vi "Convert normal string to hex string.vi"(4 "Normal String":string[](array[string])) -> (1 "Hex String":string[](array[string]))   [LabVIEW 2020]
panel:
  out "*(type *) &x 2":string
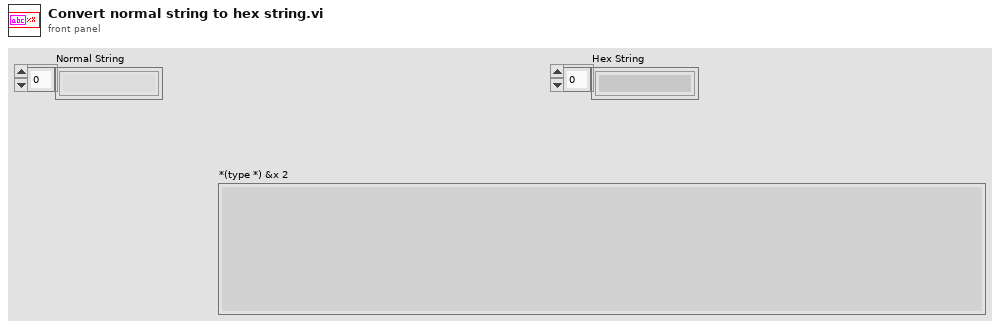
[diagram p1: front panel]
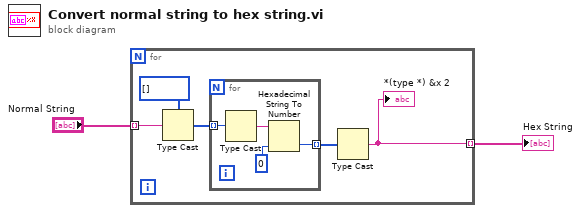
[diagram p0: block diagram]
diagram:
  n1 = for {
    tunnel: "Normal String" -> [w4] mode=indexing
    tunnel: [w3] -> w1 mode=indexing
    n2 = Type Cast(type=u16[] [], x=w4) -> (*(type *) &x=w6:u16[])
    n3 = for {
      tunnel: w6 -> [w11] mode=indexing
      tunnel: [w8] -> w5 mode=indexing
      n4 = Type Cast(x=w11) -> (*(type *) &x=w10:string)  [unwired: 1 in]
      n5 = Hexadecimal String To Number(string=w10, default (0uL)=u8 0) -> (number=w8:u8)  [unwired: 1 in, 1 out]
    }
    n6 = Type Cast(x=w5) -> (*(type *) &x=w3:string)  [unwired: 1 in]
    "*(type *) &x 2" <- w3
  }
  "Hex String" <- w1
